vi "Translate to Array Data_BU5.vi"(0 "original data":path=path "C:/Users/User/Desktop/aaa.csv", 1 "Only Use Last Value?":bool=TRUE, 2 "Electrode number, N":u16=8, 3 "Current Mode":u8[][](array[numeric]), 5 "original error":errorcluster, 7 "Array Mode":u16(ring) items=["None", "Gradient + Dipole dipole", "Gradient", "Dipole Dipole", "Schlumberger"], 9 "modified data":path=path "C:/Users/User/Desktop/test.csv", 11 "modified error":errorcluster, 12 "Inverse\nPolarity":bool=TRUE, 13 "Insert\nBreak":bool=TRUE, 14 "External\nRef":bool=TRUE) -> ()   [LabVIEW 2023]
uses:
  <vilib>/Utility/error.llb/DialogType.ctl
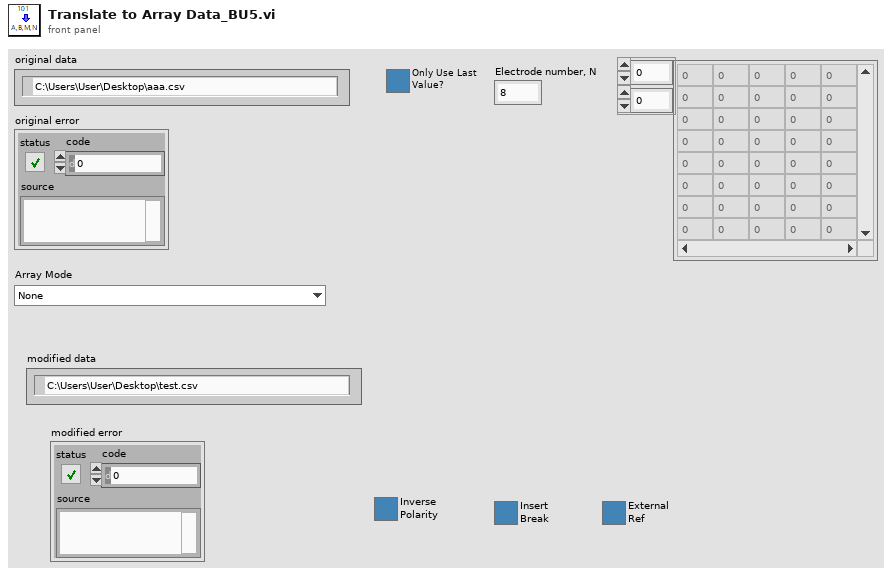
[diagram p1: front panel]
types:
  T1 = enum16{"open", "replace", "create", "open or create", "replace or create", "replace or create with confirmation"}
  T2 = typedef "DialogType.ctl" = u16
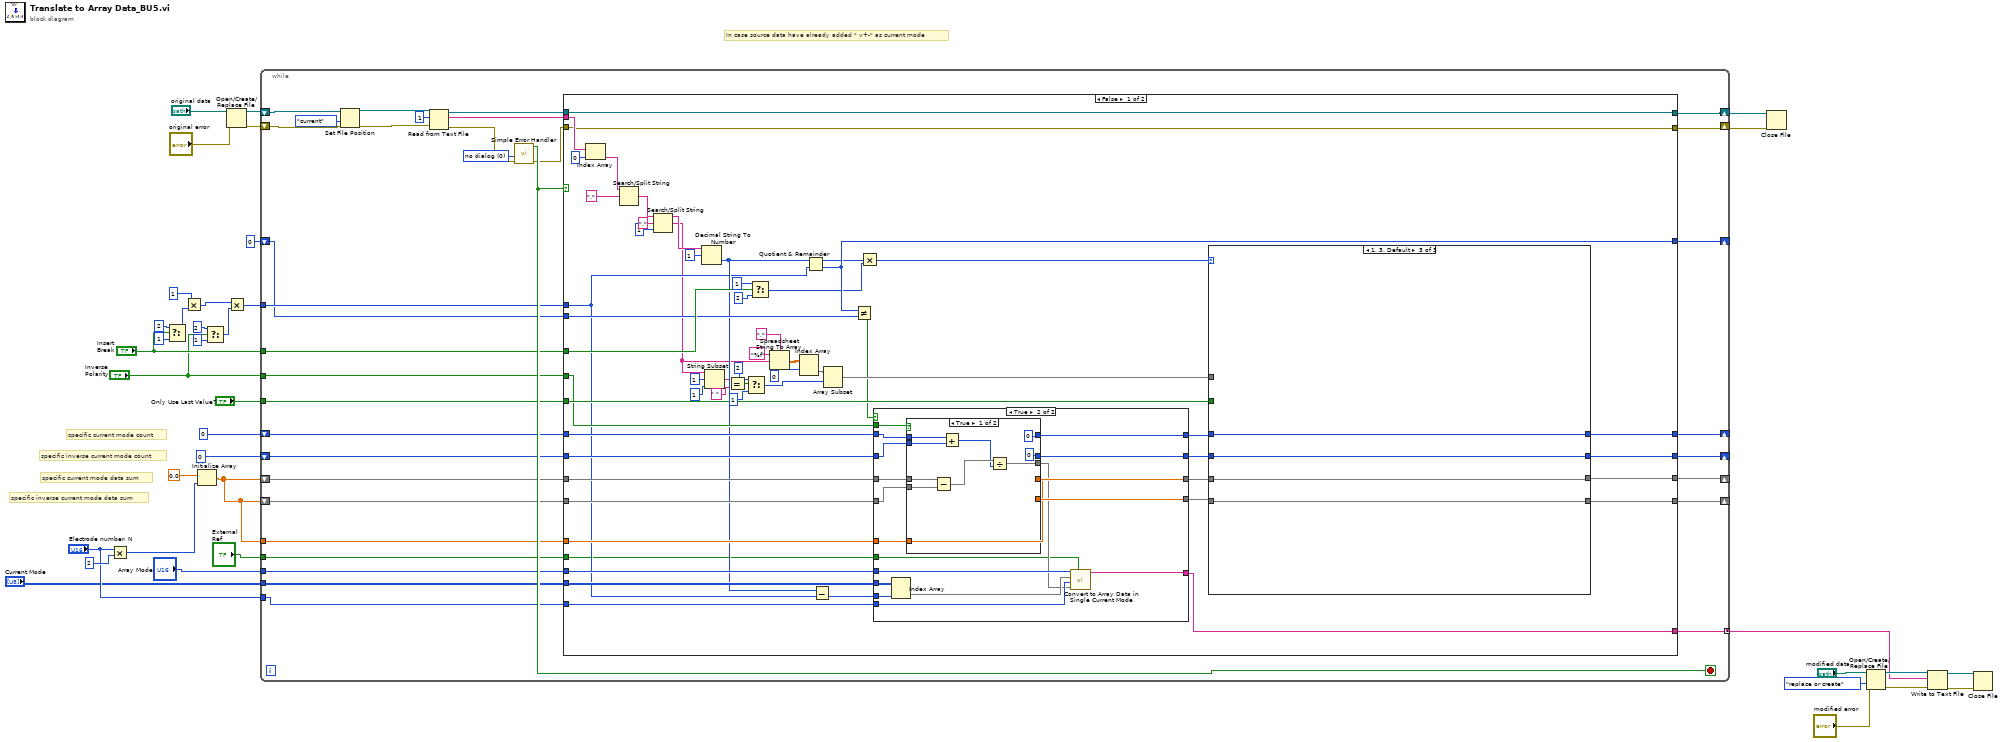
[diagram p0: block diagram]
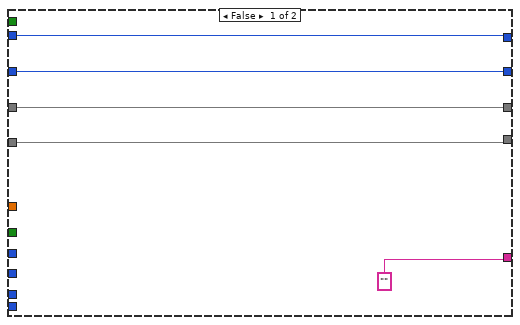
[diagram p2: hidden frame]
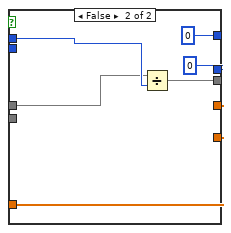
[diagram p3: hidden frame]
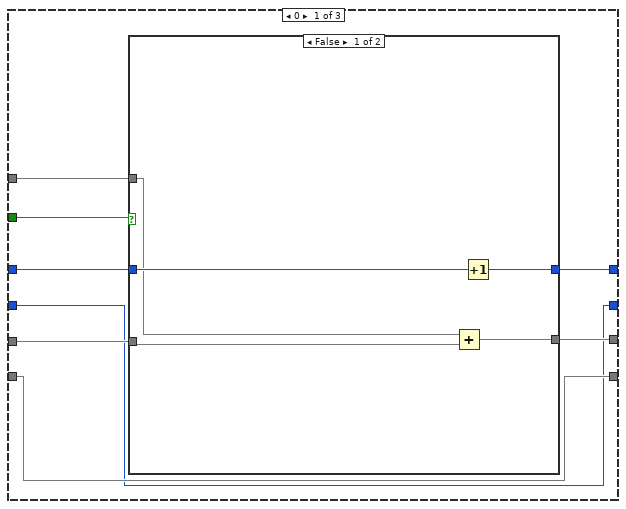
[diagram p4: hidden frame]
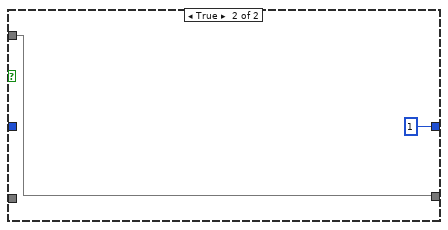
[diagram p5: hidden frame]
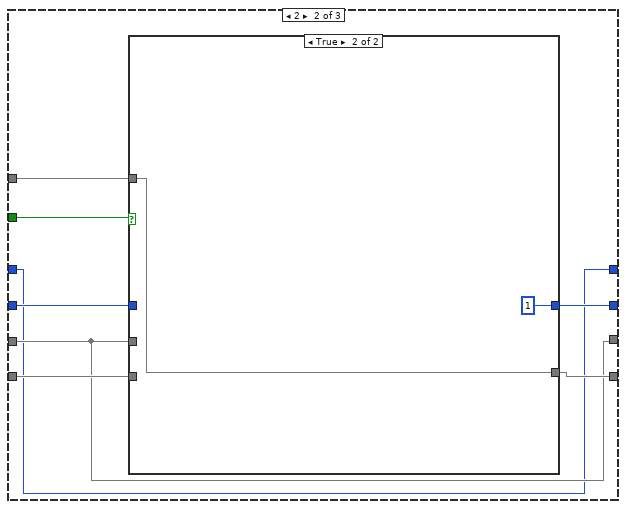
[diagram p6: hidden frame]
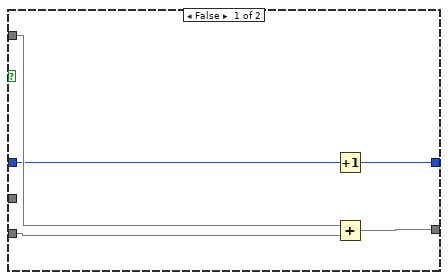
[diagram p7: hidden frame]
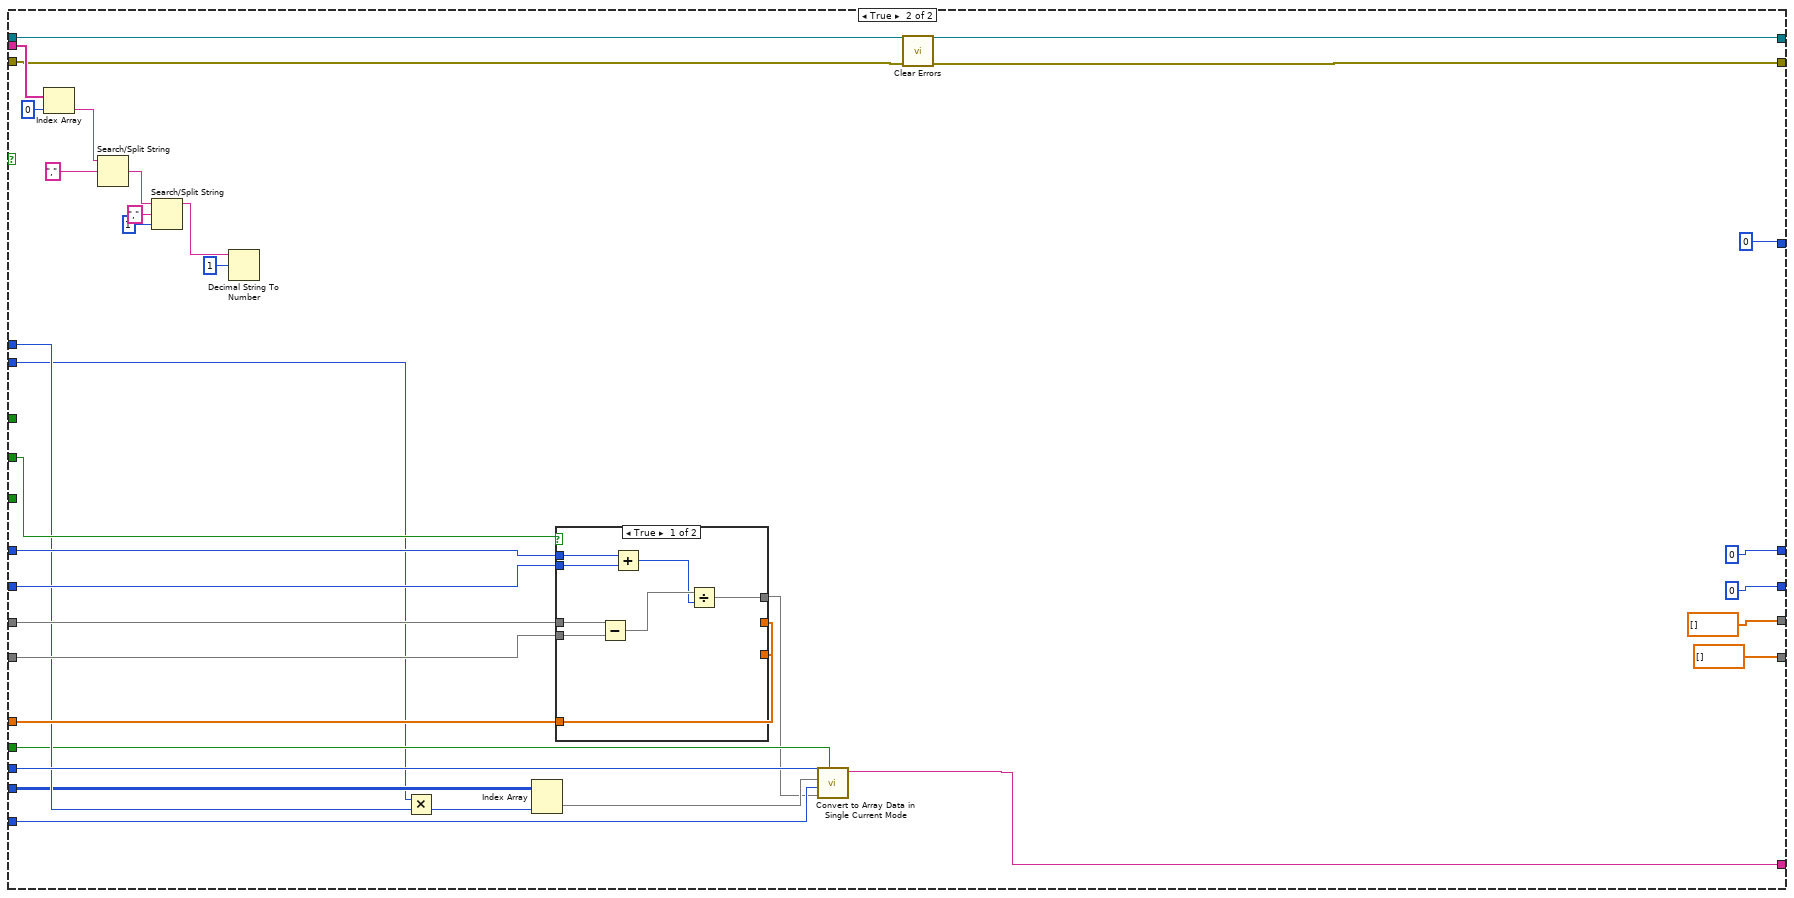
[diagram p8: hidden frame]
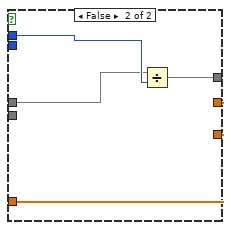
[diagram p9: hidden frame]
diagram:
  # "In case source data have already added \" v+-\" as current mode"
  # "specific inverse current mode data sum"
  # "specific current mode data sum"
  # "specific inverse current mode count"
  # "specific current mode count"
  n1 = Multiply(x="Electrode number, N", y=u16 2) -> (x*y=w11:u16)
  n2 = Select(t=2 ("number"), s="Insert\nBreak", f=1 ("number")) -> (s? t:f=w20:i32)
  n3 = Multiply(x=1 ("number"), y=w20) -> (x*y=w14:i32)
  n4 = Initialize Array(0.0 ("element"), w11) -> (w10:dbl[])
  n5 = Select(t=2 ("number"), s="Inverse\nPolarity", f=1 ("number")) -> (s? t:f=w19:i32)
  n6 = Open/Create/Replace File(file path (use dialog)="original data", error in="original error") -> (refnum out=w34:refnum<file>, error out=w35:errorcluster)  [unwired: 4 in, 1 out]
  n7 = Multiply(x=w14, y=w19) -> (x*y=w18:i32)
  n8 = while {
    shift-right: [w63] -> w29
    shift-left: w35 -> [w70]
    shift-right: [w62] -> w36
    shift-left: w34 -> [w61]
    tunnel: "Insert\nBreak" -> [w57]
    tunnel: "Inverse\nPolarity" -> [w56]
    tunnel: "Only Use Last Value?" -> [w55]
    tunnel: w18 -> [w54]
    shift-right: [w49] -> _
    shift-left: 0 ("number") -> [w53]
    shift-right: [w46] -> _
    shift-left: 0 ("number") -> [w52]
    shift-right: [w48] -> _
    shift-left: w10 -> [w51]
    shift-right: [w47] -> _
    shift-left: w10 -> [w50]
    shift-right: [w45] -> _
    shift-left: 0 -> [w44]
    tunnel: w10 -> [w43]
    tunnel: "Current Mode" -> [w41]
    tunnel: "Array Mode" -> [w42]
    tunnel: "Electrode number, N" -> [w40]
    tunnel: "External\nRef" -> [w39]
    tunnel: [w38] -> w4 mode=concatenating
    stop <- w67 stop-if-true
    w68 = T2 0 items=["no dialog", "OK message", "continue or stop message", "OK message + warnings", "continue/stop + warnings"] ("type of dialog (OK msg:1)")
    n9 = Set File Position(refnum=w61, from (0:start)=enum16{"start", "end", "current"}."current", error in=w70) -> (refnum out=w60:refnum<file>, error out=w59:errorcluster)  [unwired: 1 in]
    n10 = Read from Text File(file (use dialog)=w60, count=1, error in=w59) -> (refnum out=w65:refnum<file>, text=w66:string[], error out=w64:errorcluster)  [unwired: 1 in, 1 out]
    n11 = call <vilib>:"Simple Error Handler.vi"("type of dialog (OK msg:1)"=w68, "error in (no error)"=w64) -> ("error?"=w67:bool, "error out"=w58:errorcluster)  [unwired: 3 in, 3 out]
    n12 = case shown="False" w67 {
      tunnel: w66 -> [w125 w231]
      tunnel: w65 -> [w122 w228]
      tunnel: w58 -> [w121 w208]
      tunnel: [w122 w228] -> w62
      tunnel: [w121 w207] -> w63
      tunnel: w57 -> [w118 _]
      tunnel: w56 -> [w98 w221]
      tunnel: w55 -> [w117 _]
      tunnel: w54 -> [w84 w217]
      tunnel: w53 -> [w102 w225]
      tunnel: w52 -> [w101 w224]
      tunnel: w51 -> [w100 w223]
      tunnel: w50 -> [w99 w222]
      tunnel: [w108 0 ("number")] -> w49
      tunnel: [w107 dbl[] [] ("subarray")] -> w48
      tunnel: [w106 dbl[] [] ("subarray")] -> w47
      tunnel: [w105 0 ("number")] -> w46
      tunnel: [w103 0] -> w45
      tunnel: w44 -> [w104 w203]
      tunnel: w43 -> [w92 w220]
      tunnel: w42 -> [w88 w219]
      tunnel: w41 -> [w87 w204]
      tunnel: w40 -> [w83 w216]
      tunnel: w39 -> [w82 w215]
      tunnel: [w81 w214] -> w38
      frame False {
        n13 = Index Array(array=w125, index=0) -> (element=w123:string)
        n14 = Search/Split String(string=w123, search string/char (-)=",") -> (match + rest of string=w113:string)  [unwired: 1 in, 2 out]
        n15 = Search/Split String(string=w113, search string/char (-)=",", offset (0)=1) -> (substring before match=w114:string, match + rest of string=w73:string)  [unwired: 1 out]
        n16 = Decimal String To Number(string=w114, offset=1) -> (number=w85:i32)  [unwired: 1 in, 1 out]
        n17 = String Subset(string=w73, offset (0)=1, length (rest)=1 ("length (rest)")) -> (substring=w80:string)
        n18 = Equal?(x=w80, y=" ") -> (x = y?=w79:bool)
        n19 = Select(t=2 ("index (row)"), s=w79, f=1 ("index (row)")) -> (s? t:f=w72:i32)
        n20 = Select(t=1, s=w118, f=2 ("y")) -> (s? t:f=w91:i32)
        n21 = Spreadsheet String To Array(delimiter (Tab)=",", format string="%f", spreadsheet string=w73) -> (array=w112:dbl[][])  [unwired: 1 in]
        n22 = Index Array(array=w112, index (row)=0) -> (element=w110:dbl[])  [unwired: 1 in]
        n23 = Quotient & Remainder(x=w85, y=w84) -> (x-y*floor(x/y)=w90:i32, floor(x/y)=w103:i32)
        n24 = Subtract(x=w85, y=w84) -> (x-y=w86:i32)
        n25 = Array Subset(array=w110, index=w72) -> (w109:dbl[])  [unwired: 1 in]
        n26 = Not Equal?(x=w103, y=w104) -> (x != y?=w93:bool)
        n27 = Multiply(x=w90, y=w91) -> (x*y=w89:i32)
        n28 = case shown="True" w93 {
          tunnel: w102 -> [w134 w149]
          tunnel: w101 -> [w133 w148]
          tunnel: w100 -> [w132 w151]
          tunnel: w99 -> [w131 w150]
          tunnel: w98 -> [_ w152]
          tunnel: [w134 w147] -> w97
          tunnel: [w133 w146] -> w96
          tunnel: [w132 w145] -> w95
          tunnel: [w131 w144] -> w94
          tunnel: w92 -> [_ w143]
          tunnel: w88 -> [_ w139]
          tunnel: w87 -> [_ w142]
          tunnel: w86 -> [_ w141]
          tunnel: w83 -> [_ w138]
          tunnel: w82 -> [_ w136]
          tunnel: ["" ("String") w135] -> w81
          frame False {
          }
          frame True {
            n29 = Index Array(array=w142, index (col)=w141) -> (element=w140:u8[])  [unwired: 1 in]
            n30 = case shown="True" w152 {
              tunnel: w151 -> [w162 w165]
              tunnel: w150 -> [w161 _]
              tunnel: w149 -> [w160 w166]
              tunnel: w148 -> [w159 _]
              tunnel: [0 ("number") 0 ("number")] -> w147
              tunnel: [0 ("number") 0 ("number")] -> w146
              tunnel: [w154 w164] -> w145
              tunnel: [w154 w164] -> w144
              tunnel: w143 -> [w154 w164]
              tunnel: [w153 w163] -> w137
              frame True {
                n31 = Subtract(x=w162, y=w161) -> (x-y=w158:dbl[])
                n32 = Add(x=w160, y=w159) -> (x+y=w157:i32)
                n33 = Divide(x=w158, y=w157) -> (x/y=w153:dbl[])
              }
              frame False {
                n34 = Divide(x=w165, y=w166) -> (x/y=w163:dbl[])
              }
            }
            n35 = call "Convert to Array Data in Single Current Mode.vi"("External\nRef"=w136, "data"=w137, "Electrode number, N"=w138, "Current Mode"=w140, "Array Mode"=w139) -> ("String"=w135:string)  [unwired: 6 in]
          }
        }
        n36 = case shown="1, 3, Default" w89 {
          tunnel: w117 -> [w176 w191 _]
          tunnel: w109 -> [w172 w190 _]
          tunnel: w97 -> [w175 w184 w202]
          tunnel: w96 -> [w169 w187 w201]
          tunnel: w95 -> [w174 w185 w200]
          tunnel: w94 -> [w170 w189 w199]
          tunnel: [w173 w184 w202] -> w108
          tunnel: [w171 w185 w200] -> w107
          tunnel: [w170 w188 w199] -> w106
          tunnel: [w169 w186 w201] -> w105
          frame 0 {
            n37 = case shown="False" w176 {
              tunnel: w175 -> [w181 _]
              tunnel: w174 -> [w178 _]
              tunnel: [w180 1 ("number")] -> w173
              tunnel: w172 -> [w177 w182]
              tunnel: [w179 w182] -> w171
              frame False {
                n38 = Add(x=w177, y=w178) -> (x+y=w179:dbl[])
                n39 = Increment(x=w181) -> (x+1=w180:i32)
              }
              frame True {
              }
            }
          }
          frame 2 {
            n40 = case shown="True" w191 {
              tunnel: w185 -> [_ _]
              tunnel: w190 -> [w195 w198]
              tunnel: [w196 w198] -> w188
              tunnel: w189 -> [w194 _]
              tunnel: w187 -> [w193 _]
              tunnel: [w192 1 ("number")] -> w186
              frame False {
                n41 = Increment(x=w193) -> (x+1=w192:i32)
                n42 = Add(x=w195, y=w194) -> (x+y=w196:dbl[])
              }
              frame True {
              }
            }
          }
          frame 1, 3, Default {
          }
        }
      }
      frame True {
        n43 = Index Array(array=w231, index=0) -> (element=w229:string)
        n44 = Search/Split String(string=w229, search string/char (-)=",") -> (match + rest of string=w226:string)  [unwired: 1 in, 2 out]
        n45 = Search/Split String(string=w226, search string/char (-)=",", offset (0)=1) -> (substring before match=w227:string)  [unwired: 2 out]
        n46 = Decimal String To Number(string=w227, offset=1) -> ()  [unwired: 1 in, 2 out]
        n47 = Multiply(x=w203, y=w217) -> (x*y=w218:i32)
        n48 = Index Array(array=w204, index (col)=w218) -> (element=w206:u8[])  [unwired: 1 in]
        n49 = case shown="True" w221 {
          tunnel: w223 -> [w243 w246]
          tunnel: w222 -> [w242 _]
          tunnel: w225 -> [w241 w247]
          tunnel: w224 -> [w240 _]
          tunnel: [w237 w245] -> _
          tunnel: [w237 w245] -> _
          tunnel: w220 -> [w237 w245]
          tunnel: [w236 w244] -> w205
          frame True {
            n50 = Subtract(x=w243, y=w242) -> (x-y=w239:dbl[])
            n51 = Add(x=w241, y=w240) -> (x+y=w238:i32)
            n52 = Divide(x=w239, y=w238) -> (x/y=w236:dbl[])
          }
          frame False {
            n53 = Divide(x=w246, y=w247) -> (x/y=w244:dbl[])
          }
        }
        n54 = call "Convert to Array Data in Single Current Mode.vi"("External\nRef"=w215, "data"=w205, "Electrode number, N"=w216, "Current Mode"=w206, "Array Mode"=w219) -> ("String"=w214:string)  [unwired: 6 in]
        n55 = call <vilib>:"Clear Errors.vi"("error in (no error)"=w208) -> ("error out"=w207:errorcluster)  [unwired: 5 in, 1 out]
      }
    }
  }
  n56 = Close File(refnum=w36, error in=w29) -> ()  [unwired: 2 out]
  n57 = Open/Create/Replace File(file path (use dialog)="modified data", error in="modified error", operation (0:open)=T1."replace or create") -> (refnum out=w6:refnum<file>, error out=w5:errorcluster)  [unwired: 3 in, 1 out]
  n58 = Write to Text File(file (use dialog)=w6, text=w4, error in=w5) -> (refnum out=w3:refnum<file>, error out=w2:errorcluster)  [unwired: 1 in, 1 out]
  n59 = Close File(refnum=w3, error in=w2) -> ()  [unwired: 2 out]
